vi "AdjustVoltage.vi"(0 "object in":refnum<class "InstrumentBase.lvclass">, 2 "Desired Voltage (V)":dbl, 5 "error in (no error)":errorcluster) -> (14 "object out":refnum<class "InstrumentBase.lvclass">, 19 "error out":errorcluster)   [LabVIEW 2023, in "InstrumentBase.lvclass"]
uses:
  InstrumentBase.lvclass
  InstrumentBase.lvclass/InstrumentBase.ctl
  <vilib>/measure/matone.llb/Extract Single Tone Information 1 Chan.vi
  <vilib>/measure/NI_MAPro.lvlib
panel:
  out "AmplitudeOk":bool
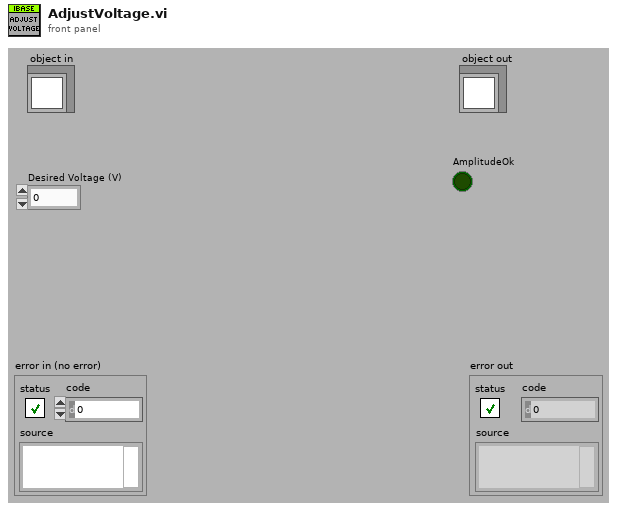
[diagram p1: front panel]
types:
  T1 = cluster{"Ch1.Carrier.Amplitude (V)":dbl, "Ch2.Carrier.Amplitude(V)":dbl}
  T2 = cluster{"Config.Ch1.Carrier.Frequency (Hz)":dbl, "Config.Ch2.Carrier.Frequency (Hz)":dbl, "Config.Ch1.Carrier.Amplitude (V)":dbl, "Config.Ch2.Carrier.Amplitude (V)":dbl}
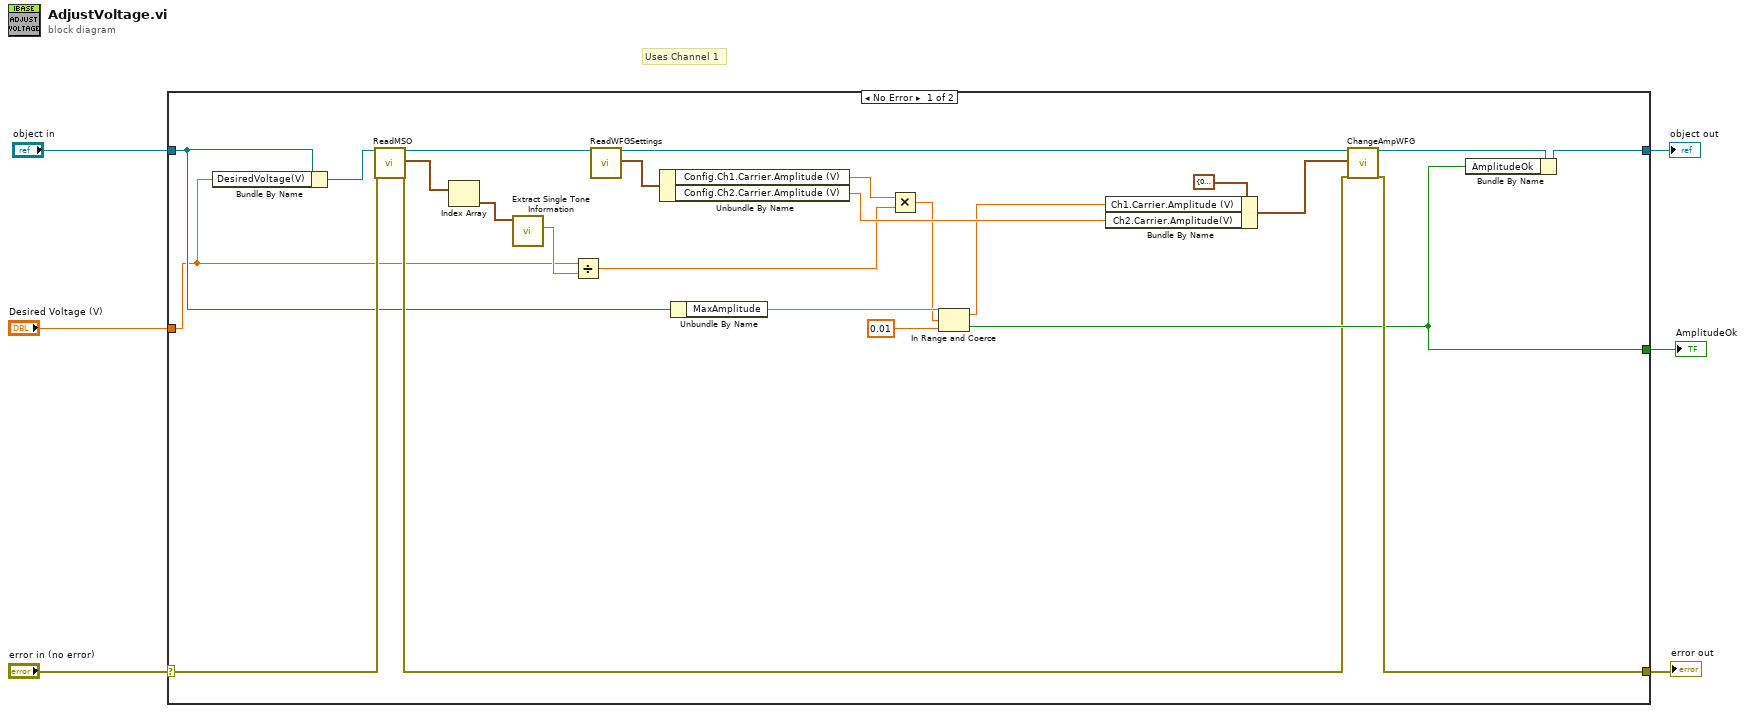
[diagram p0: block diagram]
diagram:
  # "Uses Channel 1"
  n1 = case shown="No Error" "error in (no error)" {
    selector: "error in (no error)" -> [w12 w32]
    tunnel: [w24 w32] -> w5
    tunnel: [w21 w31] -> w3
    tunnel: "object in" -> [w8 w31]
    tunnel: "Desired Voltage (V)" -> [w7 _]
    tunnel: [w18 _] -> w1
    frame No Error {
      n2 = Bundle By Name(cluster=w8, "DesiredVoltage(V)"=w7) -> (w9:refnum<class "InstrumentBase.lvclass">)
      n3 = call-dynamic "ReadMSO.vi"("object in"=w9, "error in (no error)"=w12) -> ("object out"=w17:refnum<class "InstrumentBase.lvclass">, "Channels array"=w16:waveform(dbl)[], "error out"=w11:errorcluster)  [unwired: 15 in]
      n4 = Index Array(array=w16) -> (element=w15:waveform(dbl))  [unwired: 1 in]
      n5 = call-poly <vilib>:"Extract Single Tone Information.vi"("time signal in"=w15) -> ("detected amplitude"=w14:dbl)  [unwired: 5 in, 5 out]
      n6 = Divide(x=w7, y=w14) -> (x/y=w13:dbl)
      n7 = call-dynamic "ReadWFGSettings.vi"("object in"=w17) -> ("object out"=w10:refnum<class "InstrumentBase.lvclass">, "AmplitudeAndVoltage"=w28:T2)  [unwired: 16 in, 1 out]
      n8 = Unbundle By Name(w28) -> ("Config.Ch1.Carrier.Amplitude (V)"=w29:dbl, "Config.Ch2.Carrier.Amplitude (V)"=w27:dbl)
      n9 = Unbundle By Name(w8) -> ("MaxAmplitude"=w23:dbl)
      n10 = Multiply(x=w29, y=w13) -> (x*y=w20:dbl)
      n11 = In Range and Coerce(upper limit=w23, x=w20, lower limit=0.01) -> (coerced(x)=w19:dbl, In Range?=w18:bool)
      n12 = Bundle By Name(cluster=T1 {"Ch1.Carrier.Amplitude (V)"=0.0, "Ch2.Carrier.Amplitude(V)"=0.0} ("AmplitudeCh1&2"), "Ch1.Carrier.Amplitude (V)"=w19, "Ch2.Carrier.Amplitude(V)"=w27) -> (w26:T1)
      n13 = call-dynamic "ChangeAmpWFG.vi"("object in"=w10, "AmplitudeCh1&2"=w26, "error in (no error)"=w11) -> ("object out"=w25:refnum<class "InstrumentBase.lvclass">, "error out"=w24:errorcluster)  [unwired: 15 in]
      n14 = Bundle By Name(cluster=w25, "AmplitudeOk"=w18) -> (w21:refnum<class "InstrumentBase.lvclass">)
    }
    frame Error {
    }
  }
  "error out" <- w5
  "object out" <- w3
  "AmplitudeOk" <- w1
